vi "Read Image Data From BMP File.vi"(8 "错误输入":errorcluster, 11 "文件（使用对话框）":path) -> (0 "错误输出":errorcluster, 3 "Image Data":T1)   [LabVIEW 2012, in "Picture Box Tools.lvlib" / "BMP File.lvlib"]
uses:
  BMP File.lvlib
  <vilib>/picture/picture.llb/imagedata.ctl
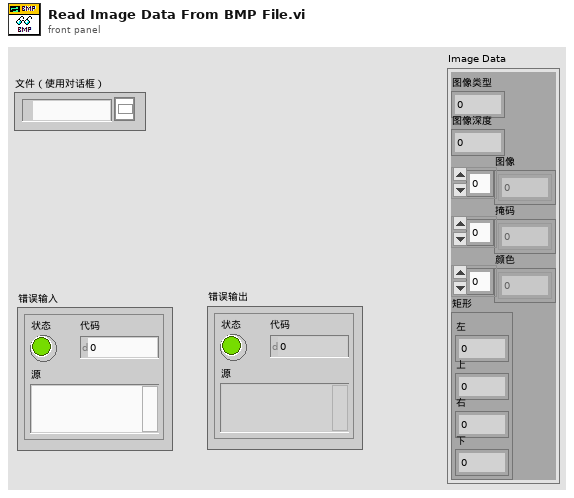
[diagram p1: front panel]
types:
  T1 = typedef "imagedata.ctl" = cluster{"image type":i32, "image depth":i32, "image":u8[], "mask":u8[], "colors":u32[], "Rectangle":cluster{"left":i16, "top":i16, "right":i16, "bottom":i16}}
  T2 = cluster{"height":u32, "width":u32, "bit depth":u16, "padded width":u32}
  T3 = typedef "Picture Box Tools.lvlib/BMP File.lvlib/Bmp Info Header.ctl" = cluster{"biSize":u32, "biWidth":i32, "biHeight":i32, "biPlanes":u16, "biBitCount":u16, "biCompression":u32, "biSizeImage":u32, "biXPelsPerMeter":i32, "biYPelsPerMeter":i32, "biCIrUsed":u32, "biCIrImportant":u32}
  T4 = cluster{"biWidth":i32, "biWidth":i32, "padded width":i32, "biHeight":i32}
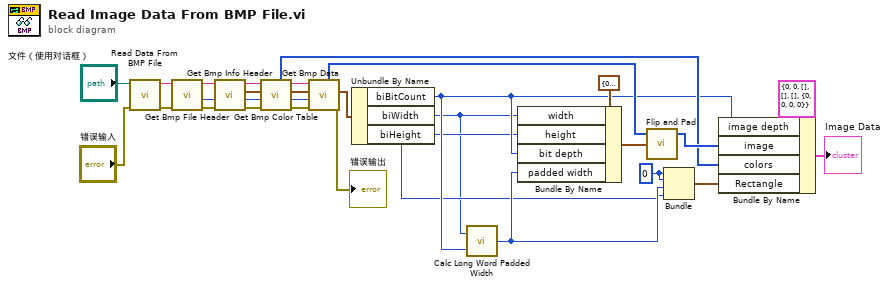
[diagram p0: block diagram]
diagram:
  w15 = 0 ("biWidth")
  n1 = call "Read Data From BMP File.vi"("错误输入"="错误输入", "文件（使用对话框）"="文件（使用对话框）") -> ("错误输出"=w29:errorcluster, "数据"=w30:string)  [unwired: 8 in]
  n2 = call "Get Bmp File Header.vi"("错误输入（无错误）"=w29, "Bmp Data In"=w30) -> ("错误输出"=w27:errorcluster, "Offset"=w26:i32, "Bmp Data Out"=w28:string)  [unwired: 6 in, 1 out]
  n3 = call "Get Bmp Info Header.vi"("错误输入"=w27, "偏移量(0)"=w26, "Bmp Data In"=w28) -> ("错误输出"=w22:errorcluster, "Offset"=w23:i32, "Info Header"=w24:T3, "Bmp Data Out"=w25:string)  [unwired: 5 in]
  n4 = call "Get Bmp Color Table.vi"("错误输入"=w22, "Offset"=w23, "Info Header In"=w24, "Bmp Data In"=w25) -> ("错误输出"=w18:errorcluster, "Offset"=w19:i32, "Info Header Out"=w20:T3, "Bmp Data Out"=w21:string, "Color Table"=w8:u32[])  [unwired: 3 in]
  n5 = call "Get Bmp Data.vi"("错误输入"=w18, "Offset"=w19, "Info Header In"=w20, "Bmp Data In"=w21) -> ("错误输出"=→"错误输出":errorcluster, "Info Header Out"=w17:T3, "Image Data"=w12:u8[])  [unwired: 5 in]
  n6 = Unbundle By Name(w17) -> ("biBitCount"=w7:u16, "biWidth"=w4:i32, "biHeight"=w5:i32)
  n7 = call "Calc Long Word Padded Width.vi"("bit depth"=w7, "width"=w4) -> ("padded width"=w6:i32)
  n8 = Bundle By Name(cluster=T2 {"height"=0, "width"=0, "bit depth"=0, "padded width"=0} ("bitmap info"), "width"=w4, "height"=w5, "bit depth"=w7, "padded width"=w6) -> (w10:T2)
  n9 = call "Flip and Pad.vi"("bitmap info"=w10, "BMP bitmap"=w12) -> ("picture bitmap"=w9:u8[])  [unwired: 3 in]
  n10 = Bundle("biWidth"=w15, "biWidth"=w15, "padded width"=w6, "biHeight"=w5) -> (w14:T4)  [unwired: 1 in]
  n11 = Bundle By Name(cluster=T1 {"image type"=0, "image depth"=0, "image"=[], "mask"=[], "colors"=[], "Rectangle"={"left"=0, "top"=0, "right"=0, "bottom"=0}} ("image data"), "image depth"=w7, "image"=w9, "colors"=w8, "Rectangle"=w14) -> (→"Image Data":T1)
